vi "Config Panel.vi"(4 "Get Config Event":refnum<user-event>, 6 "Set Config Event":refnum<user-event>, 8 "error in":errorcluster, 9 "Stop Event":refnum<user-event>, 10 "Sub Panel":refnum<vi>, 11 "Lv Proj Document Type:TAF Proj":refnum<class "TAF Proj.lvclass">) -> (0 "error out":errorcluster, 3 "Lv Proj Document Type:TAF Proj":refnum<class "TAF Proj.lvclass">)   [LabVIEW 2021, in "TAF Proj Document Type.lvlib" / "TAF Proj.lvclass"]
uses:
  <vilib>/Wovalab/AntiDoc/Document Type/Add-ons/LabVIEW TAF Project/TAF Proj/TAF Proj.lvclass
  C:/Program Files (x86)/National Instruments/LabVIEW 2021/vi.lib/Wovalab/AntiDoc/Document Type/Document/Document Type.lvclass
  <vilib>/Wovalab/AntiDoc/Document Type/Document/Config Panel Stop Argument--cluster.ctl
  <vilib>/Wovalab/AntiDoc/Document Type/Document/Config Panel Get Config Argument--cluster.ctl
  <vilib>/Wovalab/AntiDoc/Document Type/Document/Config Panel Get Config (Reply payload)--cluster.ctl
  <vilib>/Wovalab/AntiDoc/Document Type/Config/Config.lvclass
  <vilib>/Wovalab/AntiDoc/Document Type/Document/Config Panel Set Config Argument--cluster.ctl
  <vilib>/Wovalab/AntiDoc/Document Type/Document/Document Type.lvclass/Document Type.ctl
  <vilib>/Wovalab/AntiDoc/Document Type/Add-ons/LabVIEW TAF Project/TAF Proj Config/TAF Proj Config.lvclass/TAF Proj Config.ctl
  <vilib>/Wovalab/AntiDoc/Document Type/Add-ons/LabVIEW TAF Project/TAF Proj Config/TAF Proj Config.lvclass
  C:/Program Files (x86)/National Instruments/LabVIEW 2021/vi.lib/Wovalab/AntiDoc/Document Type/Config/Config.lvclass
  <vilib>/Utility/miscctls.llb/LVPointTypeDef.ctl
  <vilib>/Wovalab/AntiDoc/Document Type/Add-ons/LabVIEW TAF Project/TAF Proj Config/Write Project Path.vi
  <vilib>/Wovalab/AntiDoc/Document Type/Add-ons/LabVIEW TAF Project/TAF Proj Config/Write Document Title.vi
  <vilib>/Wovalab/AntiDoc/Document Type/Add-ons/LabVIEW TAF Project/TAF Proj Config/Write Author.vi
  <vilib>/Wovalab/AntiDoc/Document Type/Add-ons/LabVIEW TAF Project/TAF Proj Config/Write E-mail.vi
  <vilib>/Wovalab/AntiDoc/Document Type/Add-ons/LabVIEW TAF Project/TAF Proj Config/Read Project Path.vi
  <vilib>/Wovalab/AntiDoc/Document Type/Add-ons/LabVIEW TAF Project/TAF Proj Config/Read Document Title.vi
  <vilib>/Wovalab/AntiDoc/Document Type/Add-ons/LabVIEW TAF Project/TAF Proj Config/Read Author.vi
  <vilib>/Wovalab/AntiDoc/Document Type/Add-ons/LabVIEW TAF Project/TAF Proj Config/Read E-mail.vi
  <vilib>/Wovalab/AntiDoc/Document Type/Document/Read Config.vi
  <vilib>/Wovalab/AntiDoc/Document Type/Document/Write Config.vi
  <vilib>/Wovalab/AntiDoc/Document Type/Document/Document Type.lvclass
panel:
  in  "Options":bool
  in  "Email":string caption="Author e-mail:"
  in  "Author":string caption="Author name:"
  in  "Title":string caption="Document title:"
  in  "Project Path":path
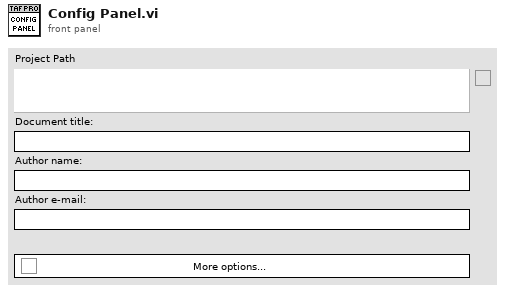
[diagram p1: front panel]
types:
  T1 = typedef "AntiDoc.lvlib/Document Type.lvclass/Config Panel Set Config Argument--cluster.ctl" = cluster{"Config":refnum<class "Config.lvclass">, "Insert Panel":bool}
  T2 = typedef "AntiDoc.lvlib/Document Type.lvclass/Config Panel Get Config (Reply payload)--cluster.ctl" = cluster{"Config":refnum<class "Config.lvclass">}
  T3 = typedef "LVPointTypeDef.ctl" = cluster{"Horizontal":i16, "Vertical":i16}
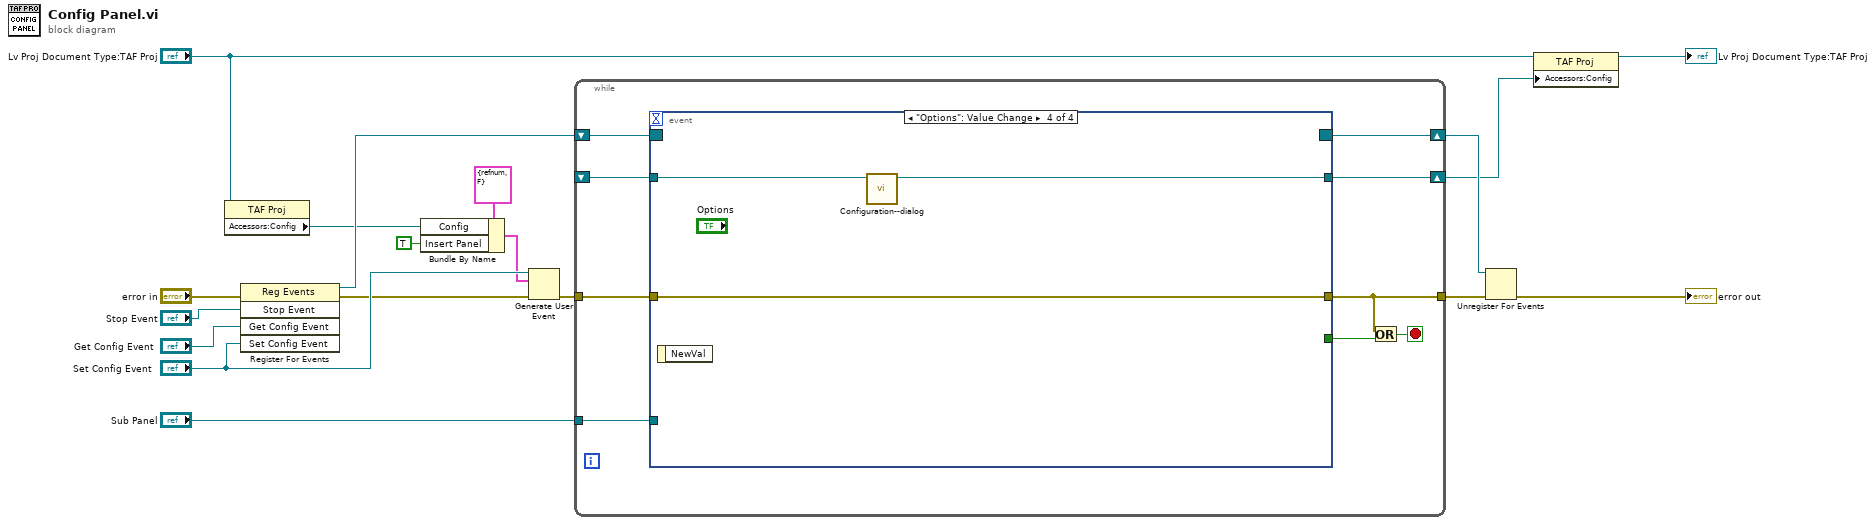
[diagram p0: block diagram]
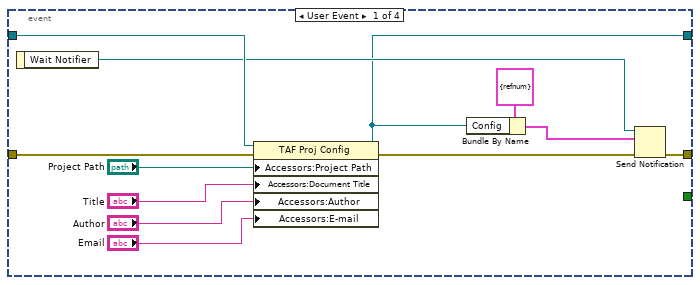
[diagram p2: hidden frame]
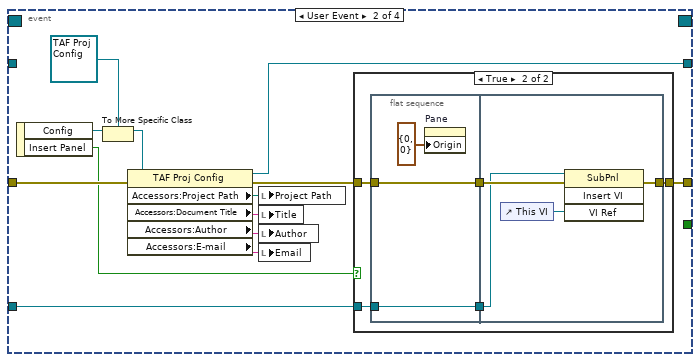
[diagram p3: hidden frame]
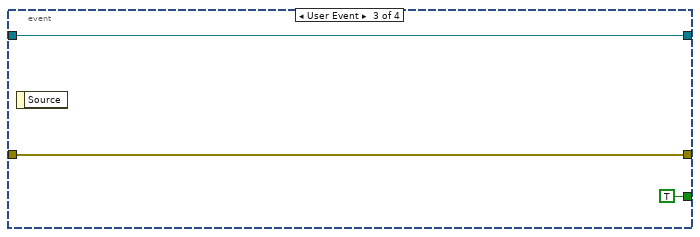
[diagram p5: hidden frame]
diagram:
  n1 = property class="TAF Proj"(reference="Lv Proj Document Type:TAF Proj") -> ("Accessors:Config"=w3:refnum<class "Config.lvclass">)  [unwired: 1 in, 2 out]
  n2 = register-events(error in="error in", "Stop Event", "Get Config Event", "Set Config Event") -> (reference out=w17:refnum<event-registration>, error out=w6:errorcluster)  [unwired: 1 in]
  n3 = Bundle By Name(cluster=T1 {"Config"=refnum, "Insert Panel"=FALSE} ("Config Panel Set config Argument"), "Config"=w3, "Insert Panel"=TRUE) -> (w4:T1)
  n4 = Generate User Event(user event="Set Config Event", event data cluster=w4, error in=w6) -> (error out=w5:errorcluster)  [unwired: 1 in, 1 out]
  n5 = while {
    tunnel: w5 -> [w25]
    tunnel: [w24] -> w13
    tunnel: "Sub Panel" -> [w19]
    shift-right: [w26] -> w14
    shift-left: w17 -> [w27]
    shift-right: [w20] -> w9
    shift-left: _ -> [w21]
    stop <- w23 stop-if-true
    n6 = event shown="[3] \"Options\": Value Change" {
      selector: w27 -> [_ _ _ _]
      dyn-events: [_ _ _ _] -> w26
      timeout: _ -> [_ _ _ _]
      tunnel: w25 -> [w36 w46 w66 w69]
      tunnel: [w31 w43 w66 w69] -> w24
      tunnel: [_ _ TRUE _] -> w22
      tunnel: w21 -> [w34 _ w68 w71]
      tunnel: [w29 w44 w68 w70] -> w20
      tunnel: w19 -> [_ w41 _ _]
      event User Event {
        n7 = event-data() -> ("Wait Notifier"=w33:refnum<notifier>)  [unwired: 1 in]
        n8 = property class="TAF Proj Config"(reference=w34, error in=w36, "Accessors:Project Path"="Project Path", "Accessors:Document Title"="Title", "Accessors:Author"="Author", "Accessors:E-mail"="Email") -> (reference out=w29:refnum<class "TAF Proj Config.lvclass">, error out=w32:errorcluster)
        n9 = Bundle By Name(cluster=T2 {"Config"=refnum} ("Get Config (Reply Payload)"), "Config"=w29) -> (w30:T2)
        n10 = Send Notification(notification=w30, notifier=w33, error in (no error)=w32) -> (error out=w31:errorcluster)  [unwired: 1 out]
      }
      event User Event {
        n11 = event-data() -> ("Config"=w51:refnum<class "Config.lvclass">, "Insert Panel"=w40:bool)  [unwired: 1 in]
        n12 = To More Specific Class(target class=refnum<class "TAF Proj Config.lvclass"> refnum ("Lv Proj Document Type.lvlib:Config"), reference=w51) -> (specific class reference=w45:refnum<class "TAF Proj Config.lvclass">)  [unwired: 1 in, 1 out]
        n13 = property class="TAF Proj Config"(reference=w45, error in=w46) -> (reference out=w44:refnum<class "TAF Proj Config.lvclass">, error out=w42:errorcluster, "Accessors:Project Path"=w50:path, "Accessors:Document Title"=w47:string, "Accessors:Author"=w49:string, "Accessors:E-mail"=w48:string)
        n14 = local write "Project Path"(w50) -> ()
        n15 = local write "Title"(w47) -> ()
        n16 = local write "Author"(w49) -> ()
        n17 = local write "Email"(w48) -> ()
        n18 = case shown="True" w40 {
          tunnel: [w53 w57] -> w43
          tunnel: w42 -> [w53 w56]
          tunnel: w41 -> [_ w54]
          frame False {
          }
          frame True {
            n19 = flat-sequence {
              tunnel: [w60] -> w58
              tunnel: w56 -> [w60]
              tunnel: [w59] -> w55
              tunnel: w54 -> [w59]
              tunnel: [w64] -> w57
              tunnel: w58 -> [w63]
              tunnel: w55 -> [w62]
              frame #0 {
                n20 = property on="Pane" class="Pane"("Origin"=T3 {"Horizontal"=0, "Vertical"=0}) -> ()  [unwired: 2 in, 2 out]
              }
              frame #1 {
                n21 = control-ref of="This VI"() -> (w65:refnum<vi>)
                n22 = invoke class="SubPnl" method="Insert VI"(reference=w62, error in=w63, "VI Ref"=w65) -> (error out=w64:errorcluster)  [unwired: 1 in, 3 out]
              }
            }
          }
        }
      }
      event User Event {
        n23 = event-data() -> ()  [unwired: 1 in, 1 out]
      }
      event "Options": Value Change {
        n24 = event-data() -> ()  [unwired: 1 in, 1 out]
        n25 = call <vilib>:"Configuration--dialog .vi"("Lv Proj Document Type:TAF Proj Config in"=w71) -> ("Lv Proj Document Type:TAF Proj Config out"=w70:refnum<class "TAF Proj Config.lvclass">)  [unwired: 10 in]
      }
    }
    n26 = Or(x=w24, y=w22) -> (x .or. y?=w23:bool)
  }
  n27 = Unregister For Events(event registration refnum=w14, error in=w13) -> (error out=→"error out":errorcluster)
  n28 = property class="TAF Proj"(reference="Lv Proj Document Type:TAF Proj", "Accessors:Config"=w9) -> (reference out=→"Lv Proj Document Type:TAF Proj":refnum<class "TAF Proj.lvclass">)  [unwired: 1 in, 1 out]
